vi "CSC_GetPtInGCS.vi"(8 "error in (no error)":errorcluster, 9 "Body ID":i32, 10 "xyz":dbl[](array[numeric])=[0.0, 0.0, 0.0], 11 "C-Alex":refnum<class "CableSerialChain.lvclass">) -> (0 "error out":errorcluster, 1 "PointVInGCS":dbl[](array[numeric]), 2 "PointInGCS":dbl[](array[numeric]), 3 "C-Alex":refnum<class "CableSerialChain.lvclass">, 4 "Point":T1={"Coord4"=[0.0, 0.0, 0.0, 1.0], "ID"=0})   [LabVIEW 2015, in "CableSerialChain.lvclass"]
uses:
  CableSerialChain.lvclass
  Body/PointOnBody.ctl
  CableSerialChain.lvclass/CableSerialChain.ctl
  <vilib>/Analysis/BLAS.llb/gemv - General Matrix-Vector Product.vi
  <vilib>/Analysis/BLAS.llb/dgemv - General Matrix-Vector Product (DBL).vi
  <vilib>/Utility/error.llb/Error Cluster From Error Code.vi
  Body/Bodies.lvclass
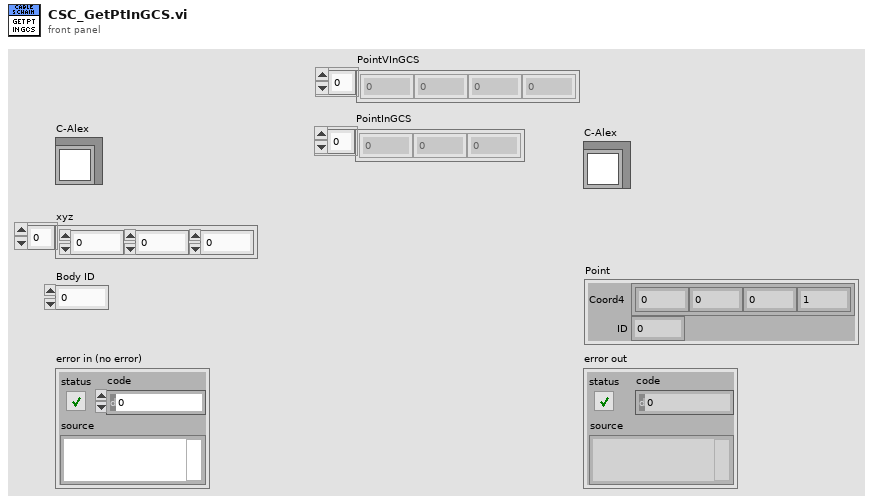
[diagram p1: front panel]
types:
  T1 = typedef "Bodies.lvclass/PointOnBody.ctl" = cluster{"Coord4":dbl[], "ID":i32}
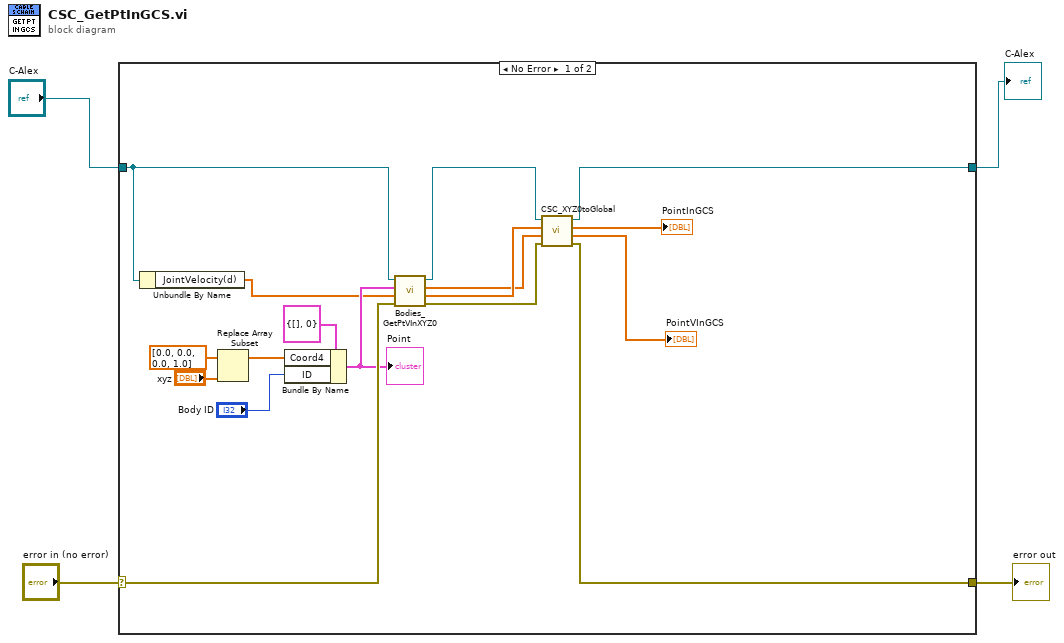
[diagram p0: block diagram]
diagram:
  n1 = case shown="No Error" "error in (no error)" {
    selector: "error in (no error)" -> [w21 w23]
    tunnel: "C-Alex" -> [w7 w22]
    tunnel: [w12 w23] -> w3
    tunnel: [w5 w22] -> w1
    frame No Error {
      n2 = Unbundle By Name(w7) -> ("JointVelocity(d)"=w9:dbl[])
      n3 = Replace Array Subset(array=dbl[] [0.0, 0.0, 0.0, 1.0] ("Coord4"), new element="xyz") -> (w15:dbl[])  [unwired: 1 in]
      n4 = Bundle By Name(cluster=T1 {"Coord4"=[], "ID"=0} ("Point"), "Coord4"=w15, "ID"="Body ID") -> (w19:T1)
      "Point" <- w19
      n5 = call "Bodies_GetPtVInXYZ0.vi"("error in (no error)"=w21, "Joint V"=w9, "Point"=w19, "Bodies.lvclass"=w7) -> ("error out"=w13:errorcluster, "Pt In GCS"=w11:dbl[], "Pt V InGCS"=w10:dbl[], "Bodies.lvclass 2"=w6:refnum<class "CableSerialChain.lvclass">)  [unwired: 4 in]
      n6 = call "CSC_XYZ0toGlobal.vi"("error in (no error)"=w13, "Vin"=w10, "Pin"=w11, "CSC In"=w6) -> ("error out"=w12:errorcluster, "Vout"=→"PointVInGCS":dbl[], "Pout"=→"PointInGCS":dbl[], "CSC Oout"=w5:refnum<class "CableSerialChain.lvclass">)  [unwired: 4 in]
    }
    frame Error {
    }
  }
  "error out" <- w3
  "C-Alex" <- w1
